vi "Close.vi"(8 "error in":errorcluster, 11 "Cfg Dev in":refnum<class "Vaisala.lvclass">=refnum) -> (0 "error out":errorcluster, 3 "Cfg Dev out":refnum<class "Vaisala.lvclass">)   [LabVIEW 2015, in "Vaisala Library.lvlib" / "Vaisala.lvclass"]
uses:
  Vaisala.lvclass
  <vilib>/MSR Consulting, LLC/General Reuse/Session APIs/_Session Fwk/Session - Root.lvclass
  <vilib>/MSR Consulting, LLC/General Reuse/Session APIs/Serial/Serial Session.lvclass
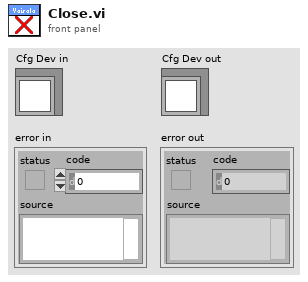
[diagram p1: front panel]
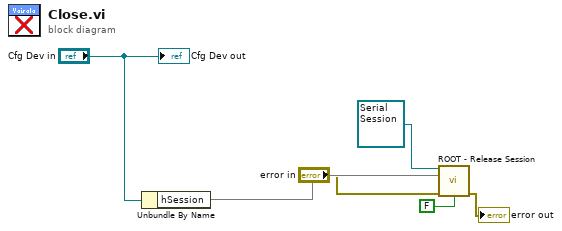
[diagram p0: block diagram]
diagram:
  n1 = Unbundle By Name("Cfg Dev in") -> ("hSession"=w5)
  n2 = call <vilib>:"ROOT - Release Session.vi"("OBJ - Session in"=refnum<class "Serial Session.lvclass"> refnum ("Serial Session"), "Session Handle in"=w5, "error in (no error)"="error in", "force destroy? (F)"=FALSE) -> ("error out"=→"error out":errorcluster)  [unwired: 10 in, 1 out]
  "Cfg Dev out" <- "Cfg Dev in"
